vi "FTPAllData.vi"() -> ()   [LabVIEW 2022 SP3]
panel:
  in  "location in":u16(ring)=3 items=["VMMC", "U_HI", "Sloan Kett", "Columbia", "RRI Test"]
  # "FTP in progress. Report errors to RRI."
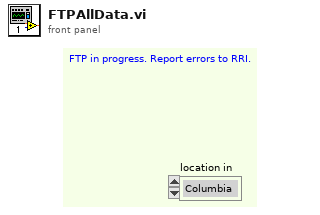
[diagram p1: front panel]
types:
  T1 = cluster{"acct":string, "passwrd":string, "ftp site":string, "subject":string, "file path":string, "recipients":string[], "SMTP Server":string}
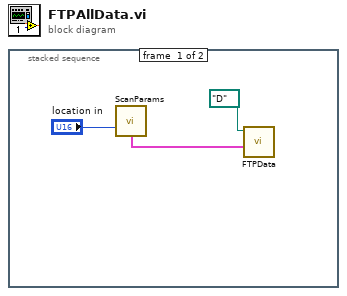
[diagram p0: block diagram]
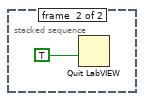
[diagram p2: hidden frame]
diagram:
  n1 = stacked-sequence {
    frame #0 {
      n2 = call "ScanParams.vi"("location in"="location in") -> ("FTP params"=w3:T1)  [unwired: 9 in, 5 out]
      n3 = call "FTPData.vi"("FTP params"=w3, "directory path"=path "D:/") -> ()  [unwired: 6 in]
    }
    frame #1 {
      n4 = Quit LabVIEW(quit? (T)=TRUE) -> ()
    }
  }
